vi "sv_Generate Waterfall View for Octave.vi"(5 "baseline":dbl format="%.2f", 6 "scale info":cluster{"x scale":dbl[], "y scale":dbl[]} {"y scale" format="%.2f"; "x scale" format="%.2f"}, 7 "clipped data":dbl[][](array[numeric]) format="%.2f", 8 "dX":dbl format="%.2f", 9 "dY":dbl format="%.2f", 10 "y scale":cluster{"y min":dbl, "y max":dbl} {"y max" format="%.2f"; "y min" format="%.2f"}, 11 "subset info":T1) -> (3 "waterfall view":cluster{dbl[], dbl[]}[](array[cluster]) {"?" format="%.2f"; "?" format="%.2f"})   [LabVIEW 2017]
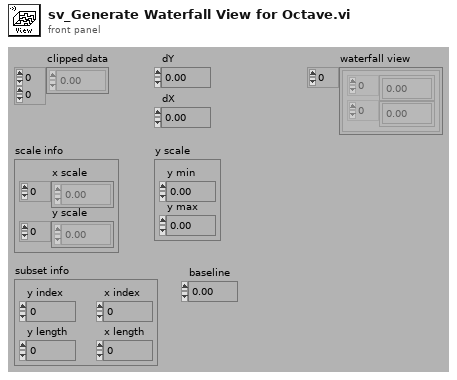
[diagram p1: front panel]
types:
  T1 = cluster{"y index":i32, "y length":i32, "x index":i32, "x length":i32}
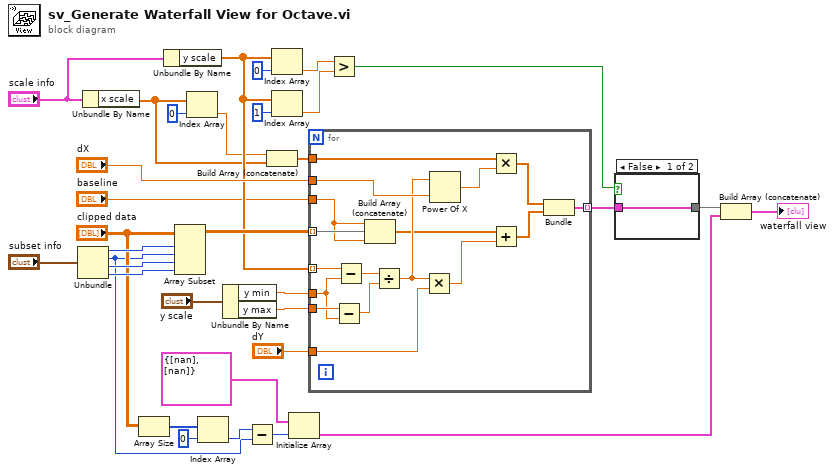
[diagram p0: block diagram]
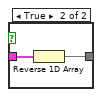
[diagram p2: hidden frame]
diagram:
  n1 = Unbundle("subset info") -> ("y index"=w25:i32, "y length"=w20:i32, "x index"=w26:i32, "x length"=w27:i32)
  n2 = Unbundle By Name("scale info") -> ("x scale"=w2:dbl[])
  n3 = Array Size(array="clipped data") -> (size(s)=w23:i32[])
  n4 = Unbundle By Name("scale info") -> ("y scale"=w7:dbl[])
  n5 = Array Subset(array="clipped data", index (row)=w25, length (row)=w20, index (col)=w26, length (col)=w27) -> (w29:dbl[][])
  n6 = Index Array(array=w2, index=0) -> (element=w3:dbl)
  n7 = Index Array(array=w23, index=0) -> (element=w21:i32)
  n8 = Unbundle By Name("y scale") -> ("y min"=w31:dbl, "y max"=w30:dbl)
  n9 = Subtract(x=w21, y=w20) -> (x-y=w19:i32)
  n10 = Build Array (concatenate)(w3, w2) -> (w4:dbl[])
  n11 = Index Array(array=w7, index=0) -> (element=w10:dbl)
  n12 = Index Array(array=w7, index=1) -> (element=w9:dbl)
  n13 = Initialize Array(cluster{dbl[], dbl[]} {[nan], [nan]} ("frame"), w19) -> (w17:cluster{dbl[], dbl[]}[])
  n14 = for {
    tunnel: w7 -> [w50] mode=indexing
    tunnel: w30 -> [w49]
    tunnel: w31 -> [w48]
    tunnel: w29 -> [w36] mode=indexing
    tunnel: w4 -> [w43]
    tunnel: "dX" -> [w39]
    tunnel: [w42] -> w14 mode=indexing
    tunnel: "dY" -> [w41]
    tunnel: "baseline" -> [w34]
    n15 = Subtract(x=w49, y=w48) -> (x-y=w46:dbl)
    n16 = Subtract(x=w50, y=w48) -> (x-y=w47:dbl)
    n17 = Build Array (concatenate)(w34, w36, w34) -> (w35:dbl[])
    n18 = Divide(x=w47, y=w46) -> (x/y=w37:dbl)
    n19 = Multiply(x=w37, y=w41) -> (x*y=w40:dbl)
    n20 = Power Of X(1:w39, 2:w37) -> (0:w38:dbl)
    n21 = Multiply(x=w43, y=w38) -> (x*y=w44:dbl[])
    n22 = Add(x=w35, y=w40) -> (x+y=w45:dbl[])
    n23 = Bundle(w44, w45) -> (w42:cluster{dbl[], dbl[]})  [unwired: 1 in]
  }
  n24 = Greater?(x=w10, y=w9) -> (0:w8:bool)
  n25 = case shown="False" w8 {
    tunnel: w14 -> [w51 w53]
    tunnel: [w51 w52] -> w13
    frame False {
    }
    frame True {
      n26 = Reverse 1D Array(array=w53) -> (reversed array=w52:cluster{dbl[], dbl[]}[])
    }
  }
  n27 = Build Array (concatenate)(w13, w17) -> (→"waterfall view":cluster{dbl[], dbl[]}[])
